vi "Sw ini read Double.vi"(3 "Error State (In)":errorcluster, 4 "Section":string, 5 "Keys":string[](array[string])=["C1a", "C1b", "C1c", "C2d"]) -> (0 "Error State (Out)":errorcluster, 1 "Multi Elements":dbl[](array[numeric]), 2 "Single Element":dbl)   [LabVIEW 2023]
uses:
  <vilib>/Utility/config.llb/Read Key (Double).vi
  <vilib>/Utility/config.llb/NI_LVConfig.lvlib
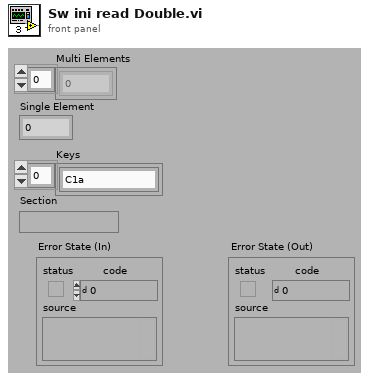
[diagram p1: front panel]
types:
  T1 = typedef "NI_LVConfig.lvlib/Config Data RefNum.ctl" = refnum<k1>
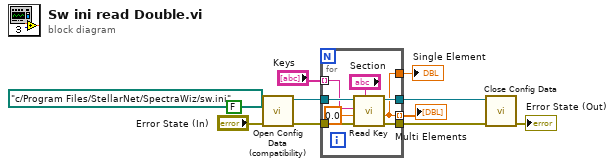
[diagram p0: block diagram]
diagram:
  n1 = call <vilib>:"Open Config Data (compatibility).vi"("error in (no error)"="Error State (In)", "create file if necessary (T)"=FALSE ("create file if necessary? (T)"), "configuration file path"=path "c:/Program Files/StellarNet/SpectraWiz/sw.ini") -> ("error out"=w9:errorcluster, "refnum"=w8:T1)  [unwired: 6 in, 1 out]
  n2 = for {
    tunnel: w9 -> [w19]
    tunnel: w8 -> [w18]
    tunnel: "Keys" -> [w17] mode=indexing
    tunnel: [w13] -> w5 mode=indexing
    tunnel: [w15] -> w7
    tunnel: [w14] -> w6
    tunnel: [w13] -> w4
    n3 = call-poly <vilib>:"Read Key.vi"("section"="Section", "error in (no error)"=w19, "default value"=0.0, "key"=w17, "refnum"=w18) -> ("error out"=w14:errorcluster, "value"=w13:dbl, "refnum out"=w15:T1)  [unwired: 3 in, 1 out]
  }
  "Multi Elements" <- w5
  "Single Element" <- w4
  n4 = call <vilib>:"Close Config Data.vi"("error in (no error)"=w6, "refnum"=w7) -> ("error out"=→"Error State (Out)":errorcluster)  [unwired: 8 in, 1 out]
